vi "Map Tag to Channel.vi"(7 "instance id":string, 8 "error in (no error)":errorcluster, 9 "Tag":string, 10 "TBM channel in":refnum<class "TBM channel.lvclass">, 11 "engine configuration in":refnum<class "engine configuration.lvclass">) -> (0 "error out":errorcluster, 3 "engine configuration out":refnum<class "engine configuration.lvclass">)   [LabVIEW 2015, in "Increment editor node.lvclass"]
uses:
  Increment editor node.lvclass
  <vilib>/NI/Tag Bus Module Framework/channel/TBM channel.lvclass
  <vilib>/NI/Module Execution Interface/Engine Configuration/engine configuration.lvclass
  <vilib>/NI/Tag Bus/tag/tag descriptor.lvclass/tag descriptor.ctl
  <vilib>/NI/Tag Bus/tag/tag descriptor.lvclass
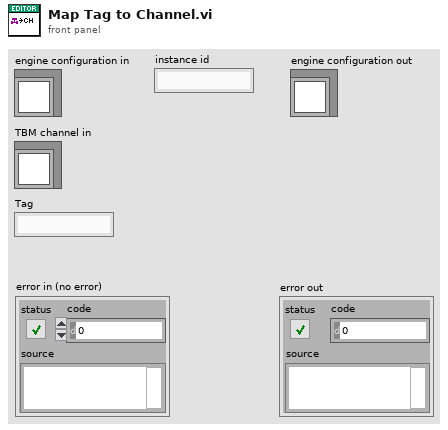
[diagram p1: front panel]
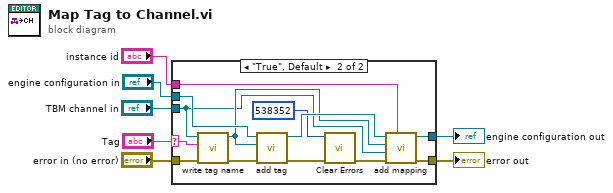
[diagram p0: block diagram]
diagram:
  n1 = case shown="\"True\", Default" "Tag" {
    selector: "Tag" -> [_ w10]
    tunnel: [w8 w21] -> w2
    tunnel: "instance id" -> [_ w20]
    tunnel: [_ w19] -> w4
    tunnel: "engine configuration in" -> [w8 w18]
    tunnel: "TBM channel in" -> [_ w15]
    tunnel: "error in (no error)" -> [_ w9]
    frame "" {
    }
    frame "True", Default {
      n2 = call <vilib>:"write tag name.vi"("error in"=w9, "name"=w10, "system tag in"=w15) -> ("error out"=w14:errorcluster, "system tag out"=w16:refnum<class "TBM channel.lvclass">)  [unwired: 7 in]
      n3 = call-dynamic "add tag.vi"("error in"=w14, "tag descriptor"=w16, "engine configuration in"=w18) -> ("error out"=w13:errorcluster, "engine configuration out"=w17:refnum<class "engine configuration.lvclass">)  [unwired: 7 in]
      n4 = call <vilib>:"Clear Errors.vi"("error in (no error)"=w13, "specific error code to clear (0: all)"=538352) -> ("error out"=w12:errorcluster)  [unwired: 4 in, 1 out]
      n5 = call-dynamic "add mapping.vi"("owner ID"=w20, "error in"=w12, "channel"=w15, "tag descriptor"=w16, "engine configuration"=w17) -> ("error out"=w19:errorcluster, "engine configuration out"=w21:refnum<class "engine configuration.lvclass">)  [unwired: 5 in]
    }
  }
  "error out" <- w4
  "engine configuration out" <- w2
